vi "WPI_MotorControlInitialize.vi"(8 "error in (no error)":errorcluster) -> (0 "error out":errorcluster, 1 "LoopTiming":u16)   [LabVIEW 2025]
doc: "This is private and only runs once. Gets an instance of the DIO object for all subsequent digital IO operations.\n\nThis software is licensed. Open the labview\\readme\\WPI Robotics Library Open Source License.txt file for more information."
uses:
  <vilib>/Rock Robotics/WPI/PWM/WPI_PWMPeriodMultiplier.ctl
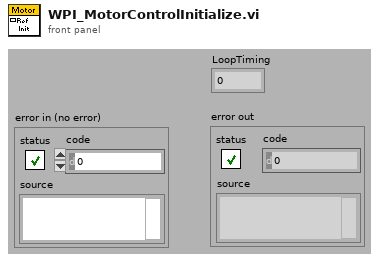
[diagram p1: front panel]
types:
  T1 = typedef "WPI_PWMPeriodMultiplier.ctl" = u8
  T2 = typedef "FPGA_DIODevRef.ctl" = cluster{"DevStatus":errorcluster}
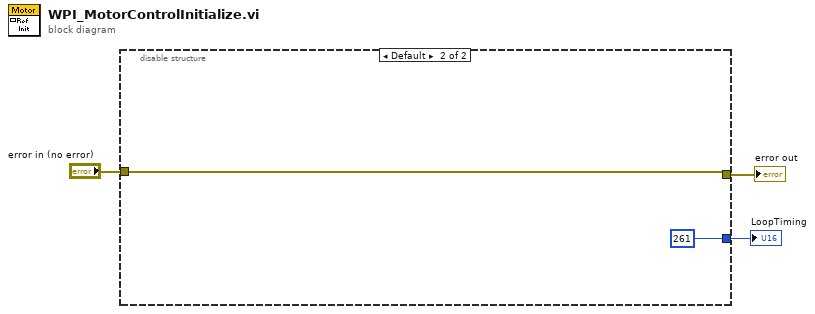
[diagram p0: block diagram]
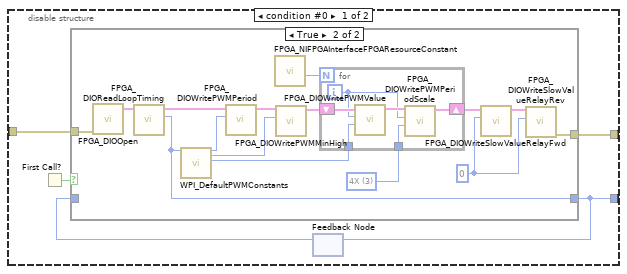
[diagram p2: hidden frame]
diagram:
  n1 = disable-structure shown="Default" {
    disable-tunnel: [w8 w33] -> w3
    disable-tunnel: [w7 261] -> w2
    disable-tunnel: "error in (no error)" -> [w4 w33]
    frame condition #0 {
      n2 = First Call?() -> (First Call?: T/F=w5:bool)
      n3 = feedback #1() -> (w6:u16)  [unwired: 1 in]
      n4 = case shown="True" w5 {
        tunnel: [w10 w17] -> w8
        tunnel: w4 -> [w10 w11]
        tunnel: [w9 w13] -> w7
        tunnel: w6 -> [w9 _]
        frame False {
        }
        frame True {
          w16 = T1 3 items=["1X"=0, "2X"=1, "4X"=3] ("PWMPeriodMultiplier")
          w21 = u8 0 ("value")
          n5 = call <vilib>:"FPGA_DIOOpen.vi"("error in (no error)"=w11) -> ("DIODeviceRef"=w12:T2)  [unwired: 1 in, 9 out]
          n6 = call <vilib>:"FPGA_DIOReadLoopTiming.vi"("DIODeviceRef In"=w12) -> ("LoopTiming"=w13:u16, "DIODeviceRef Out"=w15:T2)  [unwired: 8 in, 1 out]
          n7 = call <vilib>:"WPI_DefaultPWMConstants.vi"("DIO Loop Timing (ticks)"=w13) -> ("defaultPWMPeriod"=w20:u16, "defaultMinPWMHigh"=w19:u16, "defaultPWMDisabled"=w18:u16)  [unwired: 16 out]
          n8 = call <vilib>:"FPGA_DIOWritePWMPeriod.vi"("PWMPeriod"=w20, "DIODeviceRef In"=w15) -> ("DIODeviceRef Out"=w25:T2)  [unwired: 9 out]
          n9 = call <vilib>:"FPGA_NIFPGAInterfaceFPGAResourceConstant.vi"() -> ("NumberOfPWMs"=w24:u32)  [unwired: 11 out]
          n10 = call <vilib>:"FPGA_DIOWritePWMMinHigh.vi"("PWMMinHigh"=w19, "DIODeviceRef In"=w25) -> ("DIODeviceRef Out"=w14:T2)  [unwired: 1 in, 8 out]
          n11 = for {
            N: w24 -> [_]
            shift-right: [w29] -> w22
            shift-left: w14 -> [w31]
            tunnel: w16 -> [w27]
            tunnel: w18 -> [w26]
            i -> [w28]
            n12 = call <vilib>:"FPGA_DIOWritePWMValue.vi"("PWMValue"=w26, "PWMChannel"=w28, "DIODeviceRef In"=w31) -> ("DIODeviceRef Out"=w30:T2)  [unwired: 2 in, 6 out]
            n13 = call <vilib>:"FPGA_DIOWritePWMPeriodScale.vi"("PWMPeriodScale"=w27, "PWMChannel"=w28, "DIODeviceRef In"=w30) -> ("DIODeviceRef Out"=w29:T2)  [unwired: 1 in, 7 out]
          }
          n14 = call <vilib>:"FPGA_DIOWriteSlowValueRelayFwd.vi"("Relay Forward"=w21, "DIODeviceRef In"=w22) -> ("DIODeviceRef Out"=w23:T2)  [unwired: 1 in, 8 out]
          n15 = call <vilib>:"FPGA_DIOWriteSlowValueRelayRev.vi"("Relay Reverse"=w21, "DIODeviceRef In"=w23) -> ("error out"=w17:errorcluster)  [unwired: 1 in, 8 out]
        }
      }
      n16 = feedback-in #1(w7) -> ()
    }
    frame condition #1 (active) {
    }
  }
  "error out" <- w3
  "LoopTiming" <- w2
